vi "wait.vi"(8 "error in (no error)":errorcluster, 10 "wait (s)":dbl) -> (0 "error out":errorcluster, 2 "value out":dbl)   [LabVIEW 2017]
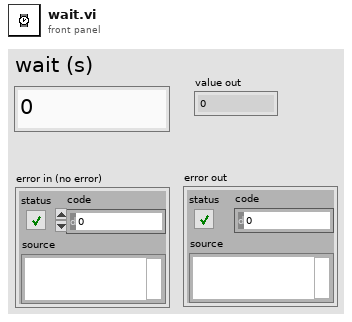
[diagram p1: front panel]
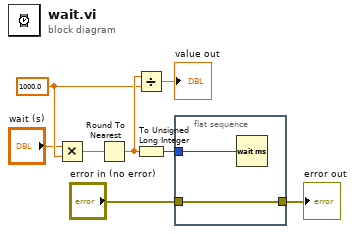
[diagram p0: block diagram]
diagram:
  w2 = 1000.0 ("y")
  n1 = Multiply(x="wait (s)", y=w2) -> (x*y=w6:dbl)
  n2 = Round To Nearest(number=w6) -> (nearest integer value=w3:dbl)
  n3 = Divide(x=w3, y=w2) -> (x/y=→"value out":dbl)
  n4 = To Unsigned Long Integer(number=w3) -> (unsigned 32bit integer=w5:u32)
  n5 = flat-sequence {
    tunnel: w5 -> [w10]
    tunnel: [w9] -> w8
    tunnel: "error in (no error)" -> [w9]
    frame #0 {
      n6 = Wait (ms)(milliseconds to wait=w10) -> ()  [unwired: 1 out]
    }
  }
  "error out" <- w8
